vi "CT-Apply Gaussian Filter.vi"(0 "Freq (Hz)":dbl, 7 "Amplitude in":dbl) -> (8 "Amplitude out":dbl)   [LabVIEW 2015]
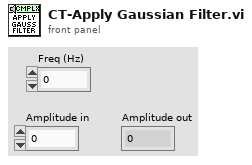
[diagram p1: front panel]
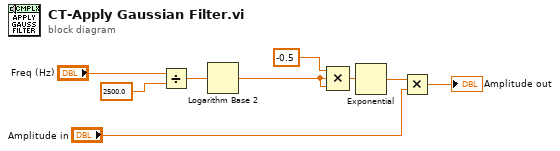
[diagram p0: block diagram]
diagram:
  n1 = Divide(x="Freq (Hz)", y=2500.0) -> (x/y=w7:dbl)
  n2 = Logarithm Base 2(1:w7) -> (0:w3:dbl)
  n3 = Compound Arithmetic op=MULTIPLY(-0.5, w3, w3) -> (w6:dbl)
  n4 = Exponential(1:w6) -> (0:w4:dbl)
  n5 = Multiply(x=w4, y="Amplitude in") -> (x*y=→"Amplitude out":dbl)
